vi "HWT_Process FGV.vi"(7 "Action":enum16{"Init", "Add", "Get"}(ring), 8 "error in (no error)":errorcluster, 11 "Queue in":refnum<queue>) -> (0 "error out":errorcluster, 3 "Queue Array out":refnum<queue>[](array[refnum]))   [LabVIEW 2015]
uses:
  Controls/Control_General Command Cluster.ctl
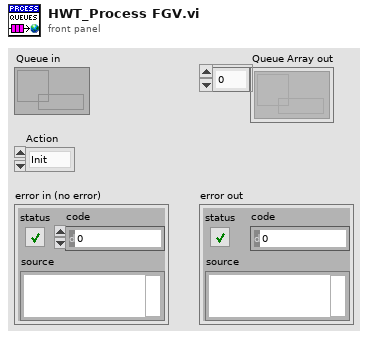
[diagram p1: front panel]
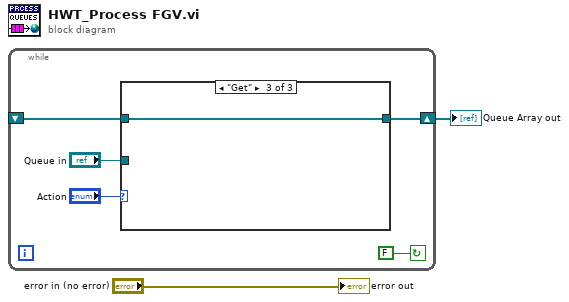
[diagram p0: block diagram]
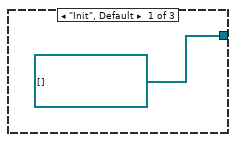
[diagram p2: hidden frame]
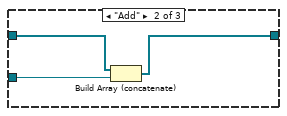
[diagram p3: hidden frame]
diagram:
  n1 = while {
    shift-right: [w5] -> w2
    shift-left: _ -> [w4]
    stop <- FALSE continue-if-true
    n2 = case shown="\"Get\"" "Action" {
      tunnel: [refnum<queue>[] [] w9 w12] -> w5
      tunnel: w4 -> [_ w10 w12]
      tunnel: "Queue in" -> [_ w11 _]
      frame "Init", Default {
      }
      frame "Add" {
        n3 = Build Array (concatenate)(w10, w11) -> (w9:refnum<queue>[])
      }
      frame "Get" {
      }
    }
  }
  "Queue Array out" <- w2
  "error out" <- "error in (no error)"
